vi "RT Host - calc intersect.vi"(7 "Current Position Global W/S Pos (mm)":dbl[](array[numeric])=[0.0, -90.0], 8 "error in (no error)":errorcluster, 10 "Previous Target Global W/S Pos (mm)":dbl[](array[numeric])=[0.0, -90.0], 11 "Target Global W/S Pos (mm)":dbl[](array[numeric])=[0.0, -90.0]) -> (0 "error out":errorcluster, 2 "Global Yint (mm)":dbl, 3 "Global Xint (mm)":dbl)   [LabVIEW 2017]
doc: "This subVI calculates the intersect of two stright perpendicular lines."
panel:
  # "Inputs"
  # "Outputs"
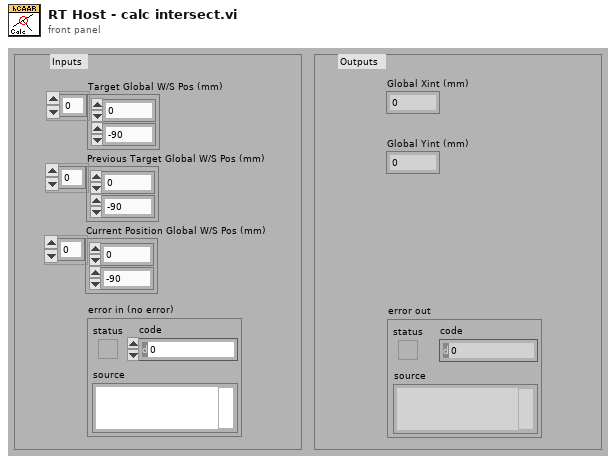
[diagram p1: front panel]
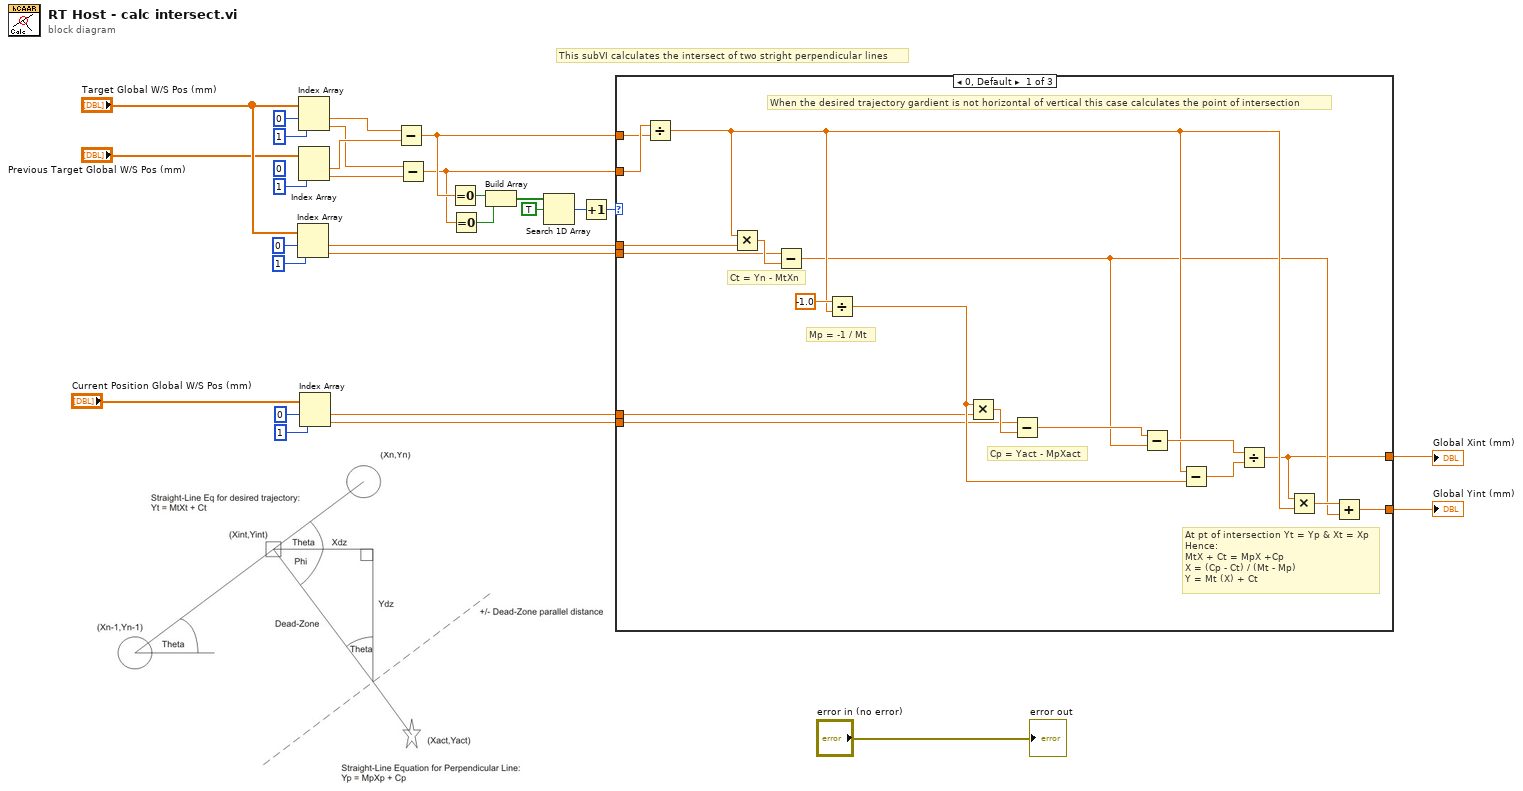
[diagram p0: block diagram]
diagram:
  (unwired) 0 ("index")
  # "This subVI calculates the intersect of two stright perpendicular lines"
  n1 = Index Array(array="Target Global W/S Pos (mm)", index #1=0 ("index"), index #2=1 ("index")) -> (element #1=w23:dbl, element #2=w22:dbl)
  n2 = Index Array(array="Target Global W/S Pos (mm)", index #1=0 ("index"), index #2=1 ("index")) -> (element #1=w18:dbl, element #2=w17:dbl)
  n3 = Index Array(array="Previous Target Global W/S Pos (mm)", index #2=1 ("index")) -> (element #1=w19:dbl, element #2=w16:dbl)  [unwired: 1 in]
  n4 = Index Array(array="Current Position Global W/S Pos (mm)", index #1=0 ("index"), index #2=1 ("index")) -> (element #1=w15:dbl, element #2=w14:dbl)
  n5 = Subtract(x=w18, y=w19) -> (x-y=w8:dbl)
  n6 = Subtract(x=w17, y=w16) -> (x-y=w7:dbl)
  n7 = Equal To 0?(x=w8) -> (x = 0?=w6:bool)
  n8 = Equal To 0?(x=w7) -> (x = 0?=w5:bool)
  n9 = Build Array(w6, w5) -> (w4:bool[])
  n10 = Search 1D Array(1D array=w4, element=TRUE) -> (index of element=w2:i32)  [unwired: 1 in]
  n11 = Increment(x=w2) -> (x+1=w1:i32)
  n12 = case shown="0, Default" w1 {
    tunnel: w7 -> [w47 _ _]
    tunnel: w8 -> [w46 _ _]
    tunnel: w23 -> [w45 w49 _]
    tunnel: w22 -> [w43 _ w50]
    tunnel: w15 -> [w33 _ w51]
    tunnel: w14 -> [w32 w48 _]
    tunnel: [w31 w49 w51] -> w10
    tunnel: [w30 w48 w50] -> w9
    frame 0, Default {
      # "When the desired trajectory gardient is not horizontal of vertical this case calculates the point of intersection"
      # "At pt of intersection Yt = Yp & Xt = Xp\nHence:\nMtX + Ct = MpX +Cp\nX = (Cp - Ct) / (Mt - Mp)\nY = Mt (X) + Ct"
      # "Cp = Yact - MpXact"
      # "Mp = -1 / Mt"
      # "Ct = Yn - MtXn"
      n13 = Divide(x=w47, y=w46) -> (x/y=w36:dbl)
      n14 = Multiply(x=w36, y=w45) -> (x*y=w44:dbl)
      n15 = Subtract(x=w43, y=w44) -> (x-y=w34:dbl)
      n16 = Divide(x=-1.0, y=w36) -> (x/y=w38:dbl)
      n17 = Multiply(x=w38, y=w33) -> (x*y=w41:dbl)
      n18 = Subtract(x=w32, y=w41) -> (x-y=w40:dbl)
      n19 = Subtract(x=w40, y=w34) -> (x-y=w39:dbl)
      n20 = Subtract(x=w36, y=w38) -> (x-y=w37:dbl)
      n21 = Divide(x=w39, y=w37) -> (x/y=w31:dbl)
      n22 = Multiply(x=w31, y=w36) -> (x*y=w35:dbl)
      n23 = Add(x=w35, y=w34) -> (x+y=w30:dbl)
    }
    frame 1 {
      # "When the desired trajectory gradient is vertical (i.e. delta X = 0) this case calculates the point of intersection"
    }
    frame 2 {
      # "When the desired trajectory gradient is horizontal (i.e. delta Y = 0) this case calculates the point of intersection"
    }
  }
  "Global Xint (mm)" <- w10
  "Global Yint (mm)" <- w9
  "error out" <- "error in (no error)"
